vi "SMTP Email Send Multiple Attachments Message.vi"(0 "smtp session":T1, 1 "attachments":T2(array[cluster]), 2 "return address":string, 3 "character set":string, 5 "recipients":string[](array[string]), 7 "subject":string, 9 "message":string, 11 "error in (no error)":errorcluster, 12 "translit":string="MacRoman iso-8859-1 macroman.trl, ToUpper iso-8859-1 toupper.trl,\nMacRomanUp MacRoman toupper.trl") -> (4 "smtp session out":T1, 6 "invalid recipients":string[](array[string]), 15 "error out":errorcluster)   [LabVIEW 2009, in "NewNI_SMTPEmail.lvlib"]
doc: "E-mails the Textual Message and multiple attachements to the Recipients using Mailserver.\n\nTextual Message: Textual message to be sent; if empty then the attachments only will be sent.\n\nAttachments: An array of clusters contaning four fields: 1) Whether it is a data stream or file; 2) If it is a data stream, then the data itself appeares in this field, otherwise the filename to get the data should be wired there; 3) Is the data textual or binary; 4) If the data is binary, what kind of data it is (e.g. application/octet-stream (default), image/jpeg, image/gif, etc.)\n\nMailserver: SMTP mailserver to be used to send the mail. Must be either specified here, or setup by using SMTP Setup.vi\n\nReturn Address: your desired return address; can be either specified here, or setup by using SMTP Setup.vi\n\nRecipients: list of mailboxes which specifiy where you want your e-mail sent.\n\nSubject: Subject of your message. Defaults to the string \"None\" if unwired.\n\nCharacter Set: the mailer provides international support. Character set value is intended for use with the foreign (non-US) character sets.\n\nInvalid Recipients: The list of recipients (out of the specified) that do not exist according to the mailserver (may not contain all the invalid recipients, especially if they are nonlocal to the SMTP server)."
uses:
  NewNI_SMTPEmail.lvlib
  SMTP Email Session.ctl
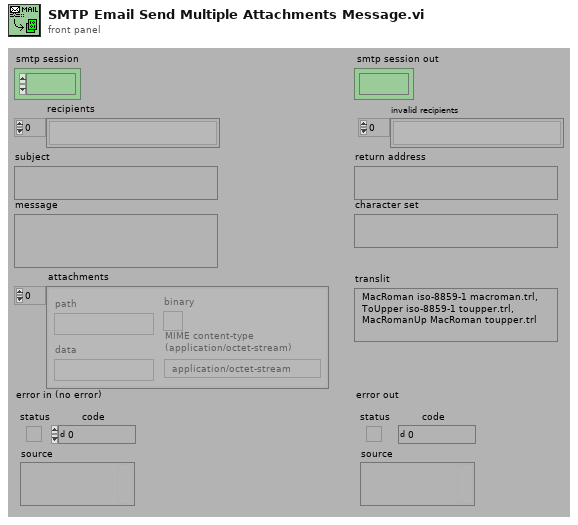
[diagram p1: front panel]
types:
  T1 = typedef "NewNI_SMTPEmail.lvlib/SMTP Email Session.ctl" = refnum<k1>
  T2 = cluster{"path":path, "data":string, "binary":bool, "MIME content-type \n(application/octet-stream)":string}[]
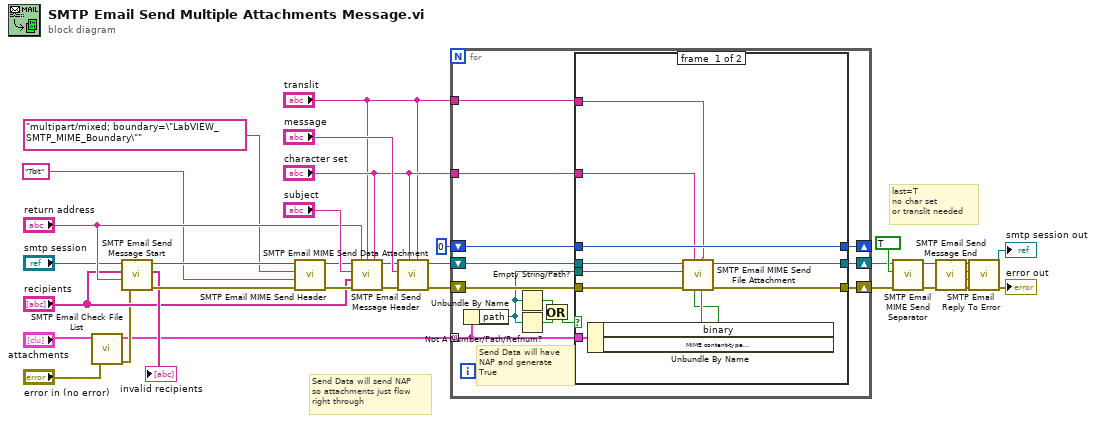
[diagram p0: block diagram]
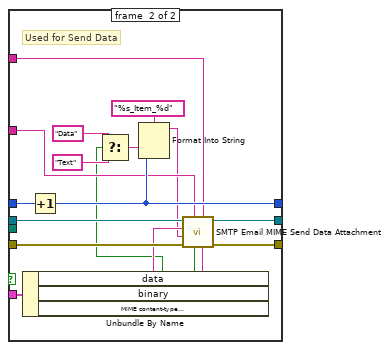
[diagram p2: hidden frame]
diagram:
  # "Send Data will send NAP\nso attachments just flow\nright through"
  # "last=T\nno char set\nor translit needed"
  n1 = call "SMTP Email Check File List.vi"("error in (no error)"="error in (no error)", "attachments"="attachments") -> ("error out"=w14:errorcluster, "attachments out"=w11:T2)  [unwired: 4 out]
  n2 = call "SMTP Email Send Message Start.vi"("error in (no error)"=w14, "return address"="return address", "recipients"="recipients", "smtp session"="smtp session") -> ("error out"=w20:errorcluster, "invalid recipients"=→"invalid recipients":string[], "smtp session out"=w21:T1)  [unwired: 1 out]
  n3 = call "SMTP Email MIME Send Header.vi"("error in (no error)"=w20, "MIME content-transfer-encoding (7bit)"="7bit", "MIME content-type (multipart/mixed)"="multipart/mixed; boundary=\"LabVIEW_SMTP_MIME_Boundary\"", "smtp session"=w21) -> ("error out"=w25:errorcluster, "smtp session out"=w26:T1)  [unwired: 2 out]
  n4 = call "SMTP Email Send Message Header.vi"("character set"="character set", "translit"="translit", "return address"="return address", "error in (no error)"=w25, "recipients"="recipients", "subject"="subject", "smtp session"=w26) -> ("error out"=w28:errorcluster, "smtp session out"=w27:T1)  [unwired: 3 out]
  n5 = call "SMTP Email MIME Send Data Attachment.vi"("translit"="translit", "character set"="character set", "error in (no error)"=w28, "data"="message", "smtp session"=w27) -> ("error out"=w22:errorcluster, "smtp session out"=w23:T1)  [unwired: 3 in, 2 out]
  n6 = for {
    tunnel: w11 -> [w47] mode=indexing
    shift-right: [w45] -> w29
    shift-left: w23 -> [w46]
    shift-right: [w41] -> w30
    shift-left: w22 -> [w42]
    shift-right: [w43] -> _
    shift-left: 0 -> [w44]
    tunnel: "character set" -> [w40]
    tunnel: "translit" -> [w35]
    # "Send Data will have\nNAP and generate\nTrue"
    n7 = Unbundle By Name(w47) -> ("path"=w39:path)
    n8 = Empty String/Path?(string/path=w39) -> (empty?=w37:bool)
    n9 = Not A Number/Path/Refnum?(number/path/refnum=w39) -> (NaN/Path/Refnum?=w38:bool)
    n10 = Or(x=w37, y=w38) -> (x .or. y?=w36:bool)
    n11 = case shown="False" w36 {
      tunnel: [w55 w70] -> w45
      tunnel: [w54 w71] -> w41
      tunnel: w46 -> [w56 w73]
      tunnel: w42 -> [w57 w72]
      tunnel: w44 -> [w58 w67]
      tunnel: [w58 w65] -> w43
      tunnel: w39 -> [w53 _]
      tunnel: w47 -> [w50 w74]
      tunnel: w40 -> [w49 w62]
      tunnel: w35 -> [w48 w59]
      frame #0 {
        n12 = Unbundle By Name(w50) -> ("binary"=w51:bool, "MIME content-type \n(application/octet-stream)"=w52:string)
        n13 = call "SMTP Email MIME Send File Attachment.vi"("MIME content-type"=w52, "translit"=w48, "binary (F)"=w51, "character set"=w49, "error in (no error)"=w57, "path"=w53, "smtp session"=w56) -> ("error out"=w54:errorcluster, "smtp session out"=w55:T1)  [unwired: 1 in, 2 out]
      }
      frame #1 {
        # "Used for Send Data"
        n14 = Unbundle By Name(w74) -> ("data"=w64:string, "binary"=w60:bool, "MIME content-type \n(application/octet-stream)"=w63:string)
        n15 = Increment(x=w67) -> (x+1=w65:i32)
        n16 = Select(t="Data", s=w60, f="Text") -> (s? t:f=w68:string)
        n17 = Format Into String(format string="%s_Item_%d", w68, w65) -> (resulting string=w61:string)  [unwired: 2 in, 1 out]
        n18 = call "SMTP Email MIME Send Data Attachment.vi"("MIME content-type"=w63, "translit"=w59, "binary (F)"=w60, "character set"=w62, "error in (no error)"=w72, "name"=w61, "data"=w64, "smtp session"=w73) -> ("error out"=w71:errorcluster, "smtp session out"=w70:T1)  [unwired: 2 out]
      }
    }
  }
  n19 = call "SMTP Email MIME Send Separator.vi"("error in (no error)"=w30, "last (F)"=TRUE, "smtp session"=w29) -> ("error out"=w17:errorcluster, "smtp session out"=w16:T1)  [unwired: 5 in, 2 out]
  n20 = call "SMTP Email Send Message End.vi"("error in (no error)"=w17, "smtp session"=w16) -> ("error out"=w10:errorcluster, "reply"=w5:string, "reply code"=w6:i32, "smtp session out"=w9:T1)  [unwired: 2 out]
  n21 = call "SMTP Email Reply To Error.vi"("error in (no error)"=w10, "reply string in"=w5, "reply code in"=w6, "smtp session"=w9) -> ("error out"=→"error out":errorcluster, "smtp session out"=→"smtp session out":T1)  [unwired: 2 out]
